vi "Calculate_(11)_Local_Cost_F()-2.vi"(0 "[IN] Cost function":i8[](array[numeric]), 1 "[IN] Subtracks":T2(array[cluster]), 3 "[IN] Still connected\ntracks in group":T1, 5 "[IN] Primary \n(X,Y) Detected":dbl[][](array[numeric]), 9 "[IN] Areas particles\nPrimary Detected":dbl[][](array[numeric]), 11 "error IN":errorcluster, 12 "[IN] Potentially\nMoving (X,Y)":dbl[][](array[numeric]), 13 "[IN] Dot matrix with statuses \nfor potentially moving dots":i16[][](array[numeric]), 14 "[IN] 3 Subsequent problem points in subtrack":bool) -> (4 "[OUT] Cost function":i8[](array[numeric]), 15 "error OUT":errorcluster)   [LabVIEW 2013]
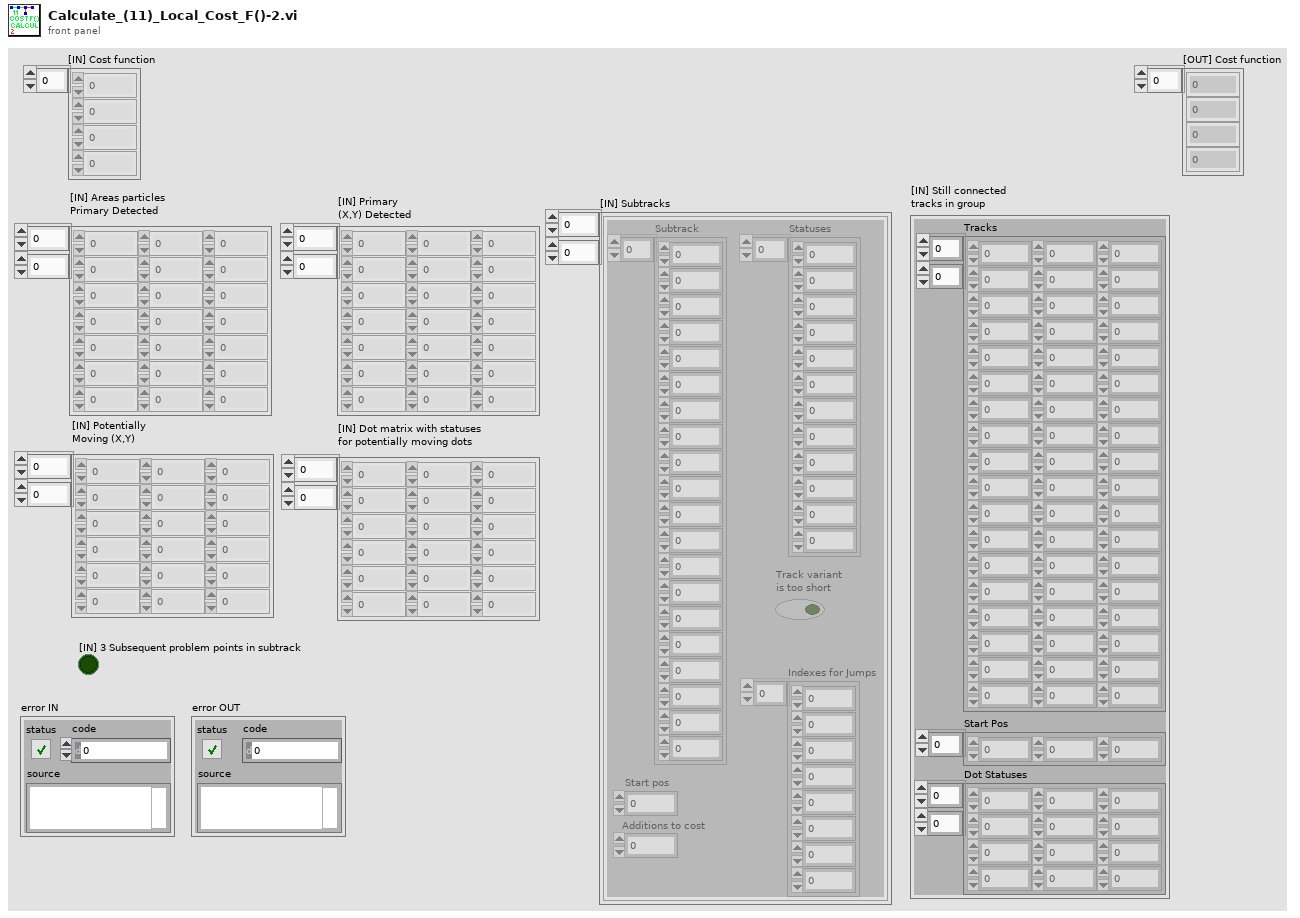
[diagram p1: front panel]
types:
  T1 = cluster{"Tracks":dbl[][], "Start Pos":i32[], "Dot Statuses":i16[][]}
  T2 = cluster{"Subtrack":dbl[], "Statuses":i16[], "Start pos":i32, "Additions to cost":i32, "Track variant \nis too short":bool, "Indexes for Jumps":i32[]}[][]
  T3 = cluster{"Subtrack":dbl[], "Statuses":i16[], "Start pos":i32, "Additions to cost":i32, "Track variant \nis too short":bool, "Indexes for Jumps":i32[]}[]
  T4 = cluster{"Subtrack":dbl[], "Statuses":i16[], "Start pos":i32, "Additions to cost":i32, "Track variant \nis too short":bool, "Indexes for Jumps":i32[]}
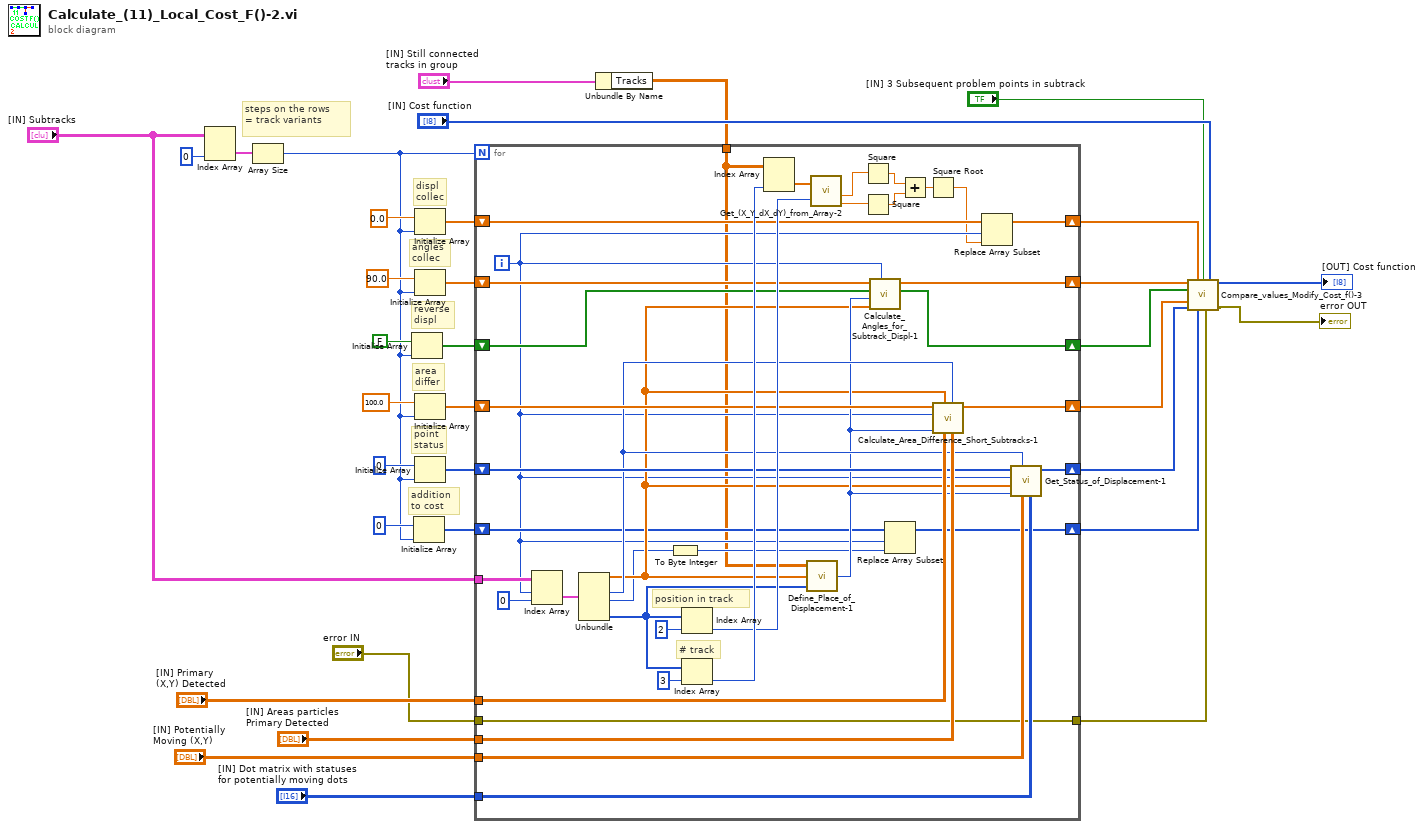
[diagram p0: block diagram]
diagram:
  # "steps on the rows\n= track variants"
  # "addition \nto cost"
  # "point\nstatus"
  # "area \ndiffer"
  # "reverse \ndispl"
  # "angles \ncollec"
  # "displ \ncollec"
  n1 = Index Array(array="[IN] Subtracks", index (col)=0 ("disabled index (col)")) -> (element=w21:T3)  [unwired: 1 in]
  n2 = Array Size(array=w21) -> (size(s)=w20:i32)
  n3 = Initialize Array(FALSE, w20) -> (w29:bool[])
  n4 = Initialize Array(i8 0, w20) -> (w23:i8[])
  n5 = Initialize Array(0.0, w20) -> (w33:dbl[])
  n6 = Initialize Array(90.0, w20) -> (w31:dbl[])
  n7 = Initialize Array(100.0, w20) -> (w27:dbl[])
  n8 = Initialize Array(i16 0, w20) -> (w25:i16[])
  n9 = Unbundle By Name("[IN] Still connected\ntracks in group") -> ("Tracks"=w1:dbl[][])
  n10 = for {
    N: w20 -> [_]
    tunnel: "[IN] Subtracks" -> [w73]
    shift-right: [w64] -> w12
    shift-left: w33 -> [w65]
    shift-right: [w61] -> w13
    shift-left: w31 -> [w62]
    shift-right: [w59] -> w9
    shift-left: w29 -> [w60]
    tunnel: "[IN] Primary \n(X,Y) Detected" -> [w55]
    tunnel: "[IN] Areas particles\nPrimary Detected" -> [w57]
    shift-right: [w56] -> w8
    shift-left: w27 -> [w58]
    tunnel: "[IN] Potentially\nMoving (X,Y)" -> [w50]
    tunnel: "[IN] Dot matrix with statuses \nfor potentially moving dots" -> [w49]
    shift-right: [w48] -> w7
    shift-left: w25 -> [w54]
    shift-right: [w43] -> w6
    shift-left: w23 -> [w47]
    tunnel: "error IN" -> [w36]
    tunnel: [w36] -> w5
    tunnel: w1 -> [w35]
    i -> [w46]
    # "# track"
    # "position in track"
    n11 = Index Array(array=w73, index (row)=w46, index (col)=0 ("disabled index (col)")) -> (element=w71:T4)
    n12 = Unbundle(w71) -> ("Subtrack"=w51:dbl[], "Start pos"=w53:i32, "Additions to cost"=w45:i32, "Indexes for Jumps"=w63:i32[])  [unwired: 2 out]
    n13 = To Byte Integer(number=w45) -> (8bit integer=w44:i8)
    n14 = Index Array(array=w63, index=2) -> (element=w66:i32)
    n15 = Index Array(array=w63, index=3) -> (element=w68:i32)
    n16 = Index Array(array=w35, index (col)=w68) -> (element=w67:dbl[])  [unwired: 1 in]
    n17 = call "Define_Place_of_Displacement-1.vi"("[IN] Indexes for Jumps"=w63, "[IN] Subtrack"=w51, "[IN] Tracks"=w35) -> ("[OUT] Index of \"11\" Dis\nplacement in Subtrack"=w52:i32)  [unwired: 2 in]
    n18 = call "Get_(X_Y_dX_dY)_from_Array-2.vi"("(X,Y,dX,dY)"=w67, "Index of Displacement"=w66) -> ("dX"=w39:dbl, "dY"=w38:dbl)  [unwired: 2 out]
    n19 = Square(x=w39) -> (x^2=w42:dbl)
    n20 = Square(x=w38) -> (x^2=w41:dbl)
    n21 = call "Calculate_Angles_for_Subtrack_Displ-1.vi"("[IN] Index of subtrack"=w46, "[IN] Subtrack"=w51, "[IN] Index of \"11\" Dis-\nplacement in Subtrack"=w52, "[IN] Reverse Displ or Not"=w60, "[IN] Array with Angles \nBetween Displacement"=w62) -> ("[OUT] Reverse displacement or not"=w59:bool[], "[OUT] Angles betwe\nen two displacements"=w61:dbl[])  [unwired: 3 in]
    n22 = Replace Array Subset(array=w47, new element=w44, index=w46) -> (w43:i8[])
    n23 = Add(x=w42, y=w41) -> (x+y=w40:dbl)
    n24 = Square Root(x=w40) -> (sqrt(x)=w37:dbl)
    n25 = call "Calculate_Area_Difference_Short_Subtracks-1.vi"("[IN] Areas particles\nPrimary Detected"=w57, "[IN] Start pos"=w53, "[IN] Primary \n(X,Y) Detected"=w55, "[IN] Subtrack"=w51, "[IN] Index of \"11\" Dis-\nplacement in Subtrack"=w52, "[IN] Index of\n subtrack"=w46, "[IN] Areas \ndifference"=w58) -> ("[OUT] Areas \ndifference"=w56:dbl[])  [unwired: 4 in]
    n26 = Replace Array Subset(array=w65, new element=w37, index=w46) -> (w64:dbl[])
    n27 = call "Get_Status_of_Displacement-1.vi"("[IN] Dot matrix with statuses\nfor potentially moving dots"=w49, "[IN] Potentially\nMoving (X,Y)"=w50, "[IN] Start pos"=w53, "[IN] Index of Problem\nPoint in Subtrack"=w52, "[IN] Subtrack"=w51, "[IN] Index of\n subtrack"=w46, "[IN] Displace-\nment Statuses"=w54) -> ("[OUT] Displace\nment Statuses"=w48:i16[])  [unwired: 4 in]
  }
  n28 = call "Compare_values_Modify_Cost_f()-3.vi"("[IN] Angles betwe\nen displacements"=w13, "[IN] Array of displa\ncement differences"=w12, "[IN] 3 Subsequent problem points in subtrack"="[IN] 3 Subsequent problem points in subtrack", "[IN] Cost function"="[IN] Cost function", "[IN] Reverse or not"=w9, "[IN] Areas \ndifferences"=w8, "[IN] Statuses of points"=w7, "[IN] Additions to cost"=w6, "error IN"=w5) -> ("[OUT] Cost function"=→"[OUT] Cost function":i8[], "error OUT"=→"error OUT":errorcluster)  [unwired: 5 in]
